vi "Spy Wait in Error.vi"(8 "error in (no error)":errorcluster, 9 "timeout in ms (-1)":i32, 11 "Mock Error Handler In":refnum<class "Mock Error Handler.lvclass">) -> (0 "error out":errorcluster, 1 "Errors":errorcluster, 2 "Location":string, 3 "Mock Error Handler Out":refnum<class "Mock Error Handler.lvclass">, 4 "Timed out?":bool)   [LabVIEW 2020, in "Mock Error Handler.lvclass"]
doc: "Spys on errors sent to the error handler. This Method requires a lock on the execution thread to prevent race conditions when testing other processes using the error handler."
uses:
  Mock Error Handler.lvclass
  Mock Error Handler.lvclass/Mock Error Handler.ctl
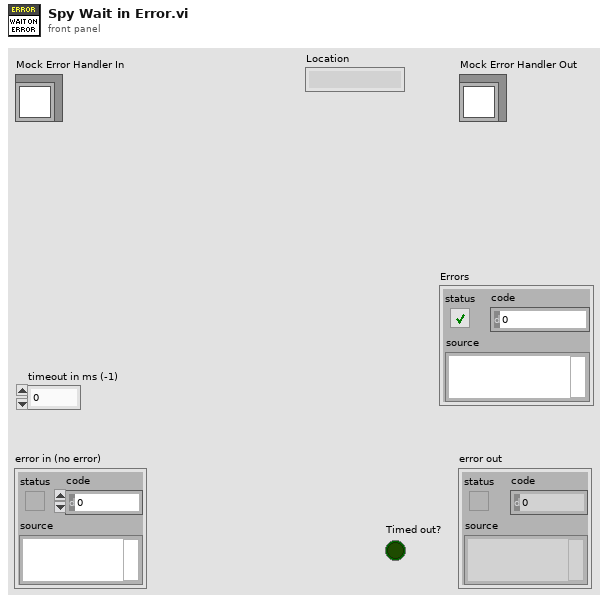
[diagram p1: front panel]
types:
  T1 = typedef "Mock Error Handler.lvclass/Error Message Data.ctl" = cluster{"Location":string, "Error":errorcluster}
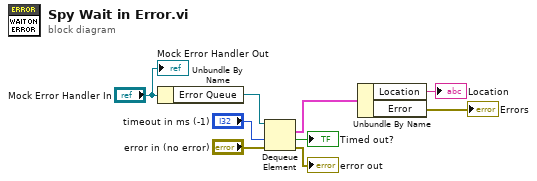
[diagram p0: block diagram]
diagram:
  n1 = Unbundle By Name("Mock Error Handler In") -> ("Error Queue"=w3:refnum<queue>)
  n2 = Dequeue Element(queue=w3, timeout in ms (-1)="timeout in ms (-1)", error in (no error)="error in (no error)") -> (element=w7:T1, timed out?=→"Timed out?":bool, error out=→"error out":errorcluster)  [unwired: 1 out]
  n3 = Unbundle By Name(w7) -> ("Location"=→"Location":string, "Error"=→"Errors":errorcluster)
  "Mock Error Handler Out" <- "Mock Error Handler In"
